vi "RT_ShVariables.vi"() -> ()   [LabVIEW 2019]
panel:
  out "StopSystem":bool
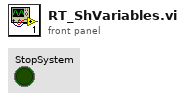
[diagram p1: front panel]
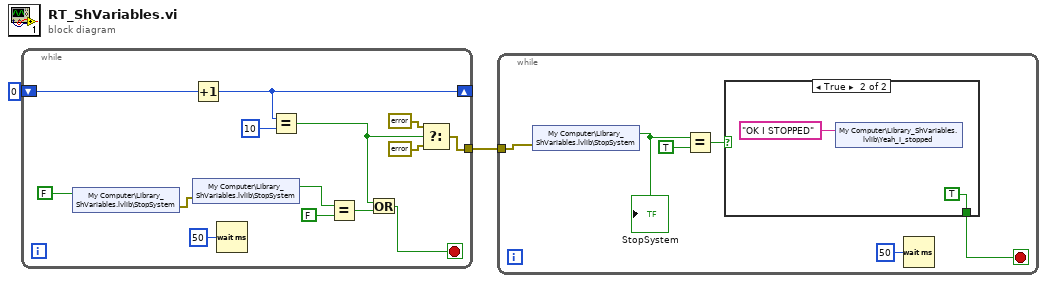
[diagram p0: block diagram]
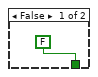
[diagram p2: hidden frame]
diagram:
  n1 = while {
    tunnel: [w8] -> w2
    shift-right: [w13] -> _
    shift-left: u8 0 -> [w14]
    stop <- w11 stop-if-true
    n2 = shared-variable "My Computer\\Library_ShVariables.lvlib\\StopSystem"(FALSE ("STOP")) -> (error out=w3:errorcluster)  [unwired: 1 in]
    n3 = Increment(x=w14) -> (x+1=w13:u8)
    n4 = shared-variable "My Computer\\Library_ShVariables.lvlib\\StopSystem"(error in=w3) -> (w4:bool)  [unwired: 1 out]
    n5 = Wait (ms)(milliseconds to wait=u32 50) -> ()  [unwired: 1 out]
    n6 = Equal?(x=w13, y=u8 10) -> (x = y?=w9:bool)
    n7 = Equal?(x=w4, y=FALSE) -> (x = y?=w10:bool)
    n8 = Or(x=w9, y=w10) -> (x .or. y?=w11:bool)
    n9 = Select(t=errorcluster {"status"=TRUE, "code"=0, "source"=""} ("error IO"), s=w9, f=errorcluster {"status"=FALSE, "code"=0, "source"=""} ("error IO")) -> (s? t:f=w8:errorcluster)
  }
  n10 = while {
    tunnel: w2 -> [w17]
    stop <- w20 stop-if-true
    n11 = shared-variable "My Computer\\Library_ShVariables.lvlib\\StopSystem"(error in=w17) -> (w18:bool)  [unwired: 1 out]
    "StopSystem" <- w18
    n12 = Equal?(x=w18, y=TRUE) -> (x = y?=w21:bool)
    n13 = case shown="True" w21 {
      tunnel: [FALSE TRUE] -> w20
      frame False {
      }
      frame True {
        n14 = shared-variable "My Computer\\Library_ShVariables.lvlib\\Yeah_I_stopped"("OK I STOPPED" ("Yeah_I_stopped")) -> ()  [unwired: 1 in, 1 out]
      }
    }
    n15 = Wait (ms)(milliseconds to wait=u32 50) -> ()  [unwired: 1 out]
  }
